vi "Execute Python Optimization (On-Grid).vi"(6 "Results Queue":refnum<queue>, 8 "error in":errorcluster, 11 "On-Grid in":refnum<class "On-Grid.lvclass">) -> (0 "error out":errorcluster, 3 "On-Grid out":refnum<class "On-Grid.lvclass">)   [LabVIEW 2018, in "On-Grid Actor.lvlib" / "On-Grid.lvclass"]
uses:
  On-Grid.lvclass
  C:/Users/Administrator/Desktop/LabVIEW EMS/Optimization/Generic Optimization Actor/Generic Optimization/Generic Optimization.lvclass
  Generic Optimization Actor/Generic Optimization/Controls/Grid State for Optimization.ctl
  Global Variables/Global Variables.vi
  Generic Optimization Actor/Generic Optimization/Generic Optimization.lvclass
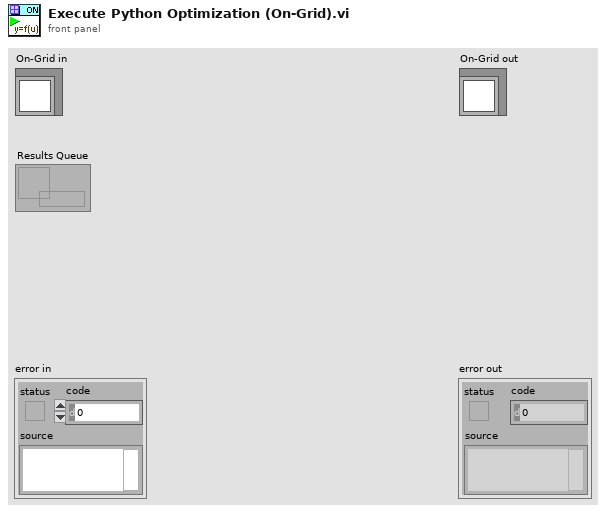
[diagram p1: front panel]
types:
  T1 = typedef "Generic Optimization Actor.lvlib/Generic Optimization.lvclass/Grid State for Optimization.ctl" = enum16{"Invalid", "On-Grid", "Off-Grid", "Island", "Resynch", "Blackstart", "Networked"}
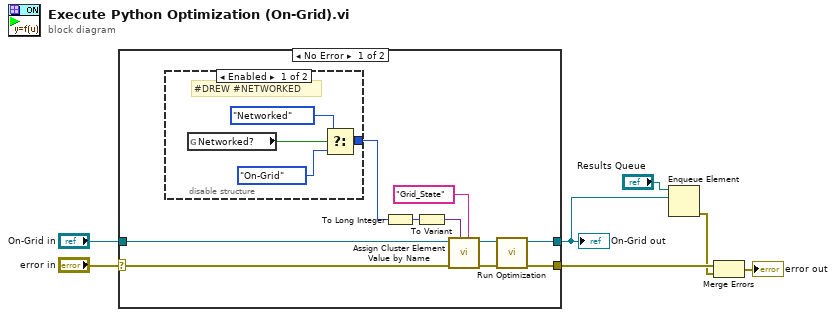
[diagram p0: block diagram]
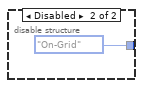
[diagram p2: hidden frame]
diagram:
  n1 = case shown="No Error" "error in" {
    selector: "error in" -> [w14 w24]
    tunnel: [w10 w24] -> w3
    tunnel: [w8 w23] -> w4
    tunnel: "On-Grid in" -> [w12 w23]
    frame No Error {
      n2 = disable-structure shown="Enabled" {
        disable-tunnel: [w19 Grid_State_for_Optimization."On-Grid"] -> w13
        frame Enabled {
          # "#DREW #NETWORKED"
          n3 = global read "Global Variables.vi" "Networked?"() -> (w21:bool)
          n4 = Select(t=Grid_State_for_Optimization."Networked", s=w21, f=Grid_State_for_Optimization."On-Grid") -> (s? t:f=w19:T1)
        }
        frame Disabled {
        }
      }
      n5 = To Long Integer(number=w13) -> (32bit integer=w15:i32)
      n6 = To Variant(anything=w15) -> (Variant=w16:variant)
      n7 = call "Assign Cluster Element Value by Name.vi"("Element Name"="Grid_State" ("Keyword Name"), "Value"=w16, "error in"=w14, "Generic Optimization"=w12) -> ("error out"=w11:errorcluster, "Generic Optimization out"=w9:refnum<class "On-Grid.lvclass">)  [unwired: 6 in]
      n8 = call "Run Optimization.vi"("error in"=w11, "Generic Optimization"=w9) -> ("error out"=w10:errorcluster, "Generic Optimization out"=w8:refnum<class "On-Grid.lvclass">)  [unwired: 8 in]
    }
    frame Error {
    }
  }
  "On-Grid out" <- w4
  n9 = Enqueue Element(queue="Results Queue", element=w4) -> (error out=w1:errorcluster)  [unwired: 2 in, 2 out]
  n10 = Merge Errors(w3, w1) -> (→"error out":errorcluster)
